vi "Air Viscosity.vi"(11 "Temperature (K)":dbl) -> (3 "Viscosity (Pa-s)":dbl)   [LabVIEW 2019]
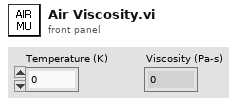
[diagram p1: front panel]
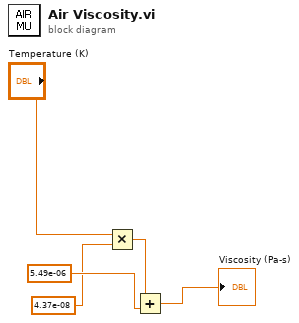
[diagram p0: block diagram]
diagram:
  n1 = Multiply(x="Temperature (K)", y=4.37e-08) -> (x*y=w4:dbl)
  n2 = Add(x=w4, y=5.49e-06) -> (x+y=→"Viscosity (Pa-s)":dbl)
